vi "Subscribe (SingleTopic).vi"(8 "error in (no error)":errorcluster, 9 "QoS":T1, 10 "Topic Filter":string, 11 "MQTT_Base in":refnum<class "MQTT_Base.lvclass">) -> (0 "error out":errorcluster, 3 "MQTT_Base out":refnum<class "MQTT_Base.lvclass">)   [LabVIEW 2013, in "MQTT Server.lvlib" / "MQTT_Base.lvclass"]
uses:
  MQTT_Base.lvclass
  Control Packets/ControlPacket/QualityOfService -- enum.ctl
  Control Packets/SUBSCRIBE/Topic Subscription -- cluster.ctl
  Control Packets/SUBSCRIBE/SUBSCRIBE.lvclass
  Control Packets/ControlPacket/ControlPacket.lvclass
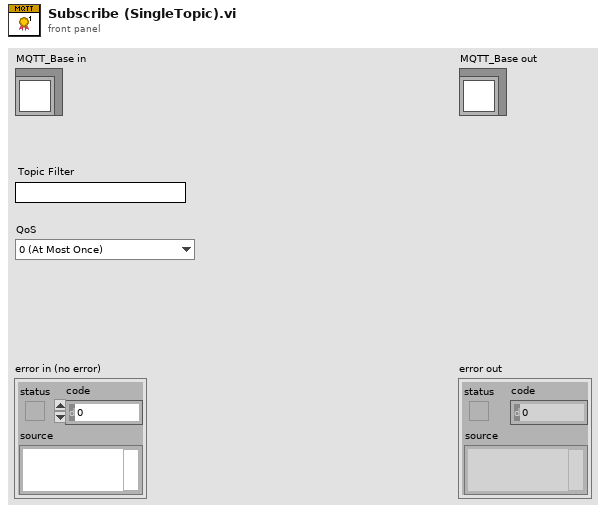
[diagram p1: front panel]
types:
  T1 = typedef "ControlPacket.lvclass/QualityOfService -- enum.ctl" = enum16{"0 (At Most Once)", "1 (At Least Once)", "2 (Exactly Once)"}
  T2 = typedef "SUBSCRIBE.lvclass/Topic Subscription -- cluster.ctl" = cluster{"Topic Filter":string, "QoS":T1}
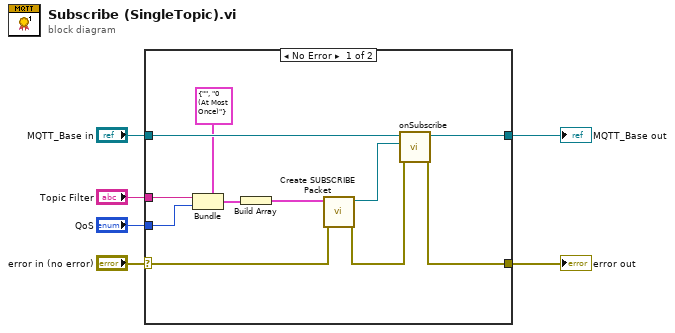
[diagram p0: block diagram]
diagram:
  n1 = case shown="No Error" "error in (no error)" {
    selector: "error in (no error)" -> [w12 w19]
    tunnel: [w15 w19] -> w5
    tunnel: [w16 w18] -> w3
    tunnel: "MQTT_Base in" -> [w17 w18]
    tunnel: "Topic Filter" -> [w11 _]
    tunnel: "QoS" -> [w10 _]
    frame No Error {
      n2 = Bundle(cluster=T2 {"Topic Filter"="", "QoS"=enum."0 (At Most Once)"} ("Topic Subscription"), "Topic Filter"=w11, "QoS"=w10) -> (w9:T2)
      n3 = Build Array(w9) -> (w8:T2[])
      n4 = call "Create SUBSCRIBE Packet.vi"("error in (no error)"=w12, "Topic Subscriptions"=w8) -> ("error out"=w13:errorcluster, "SUBSCRIBE out"=w14:refnum<class "SUBSCRIBE.lvclass">)  [unwired: 8 in]
      n5 = call-dynamic "onSubscribe.vi"("error in (no error)"=w13, "SUBSCRIBE"=w14, "MQTT_Base in"=w17) -> ("error out"=w15:errorcluster, "MQTT_Base out"=w16:refnum<class "MQTT_Base.lvclass">)  [unwired: 6 in, 1 out]
    }
    frame Error {
    }
  }
  "error out" <- w5
  "MQTT_Base out" <- w3
